vi "class_data.vi"() -> ()   [LabVIEW 2010, in "GenericAnalyser.lvclass"]
uses:
  GenericAnalyser.lvclass
panel:
  in  "latest instance":refnum<class "GenericAnalyser.lvclass">
  in  "locked by":string
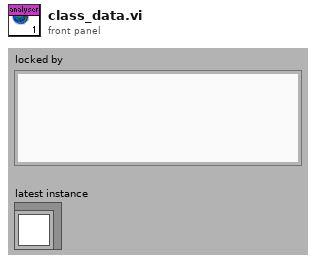
[diagram p1: front panel]
diagram:
